vi "Read Current LogicOut Statuses.vi"(11 "VacuumLines in":refnum<class "VacuumLines.lvclass">) -> (2 "Current LogicOut Statuses":bool[](array[boolean]), 3 "VacuumLines out":refnum<class "VacuumLines.lvclass">)   [LabVIEW 2016, in "Hardware.lvlib" / "VacuumLine.lvlib" / "VacuumLines.lvclass"]
uses:
  <userlib>/Common Components/Hardware/Abstract System/VacuumLine/VacuumLines/VacuumLines.lvclass
  <userlib>/Common Components/Hardware/Abstract System/VacuumLine/VacuumLines/VacuumLines.lvclass/VacuumLines.ctl
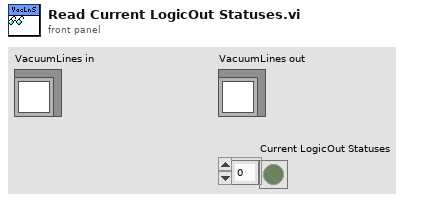
[diagram p1: front panel]
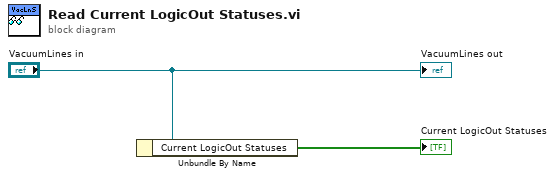
[diagram p0: block diagram]
diagram:
  n1 = Unbundle By Name("VacuumLines in") -> ("Current LogicOut Statuses"=→"Current LogicOut Statuses":bool[])
  "VacuumLines out" <- "VacuumLines in"
